vi "AI_StreamingAI_Save_Read.vi"() -> ()   [LabVIEW 2012]
panel:
  out "overrun count":i32
  in  "read buffer size":u64=131072
  in  "convert rate":dbl=1000000.0
  in  "channel count":i32=2
  in  "y min":dbl
  in  "y max":dbl=10.0
  in  "time out(s)":i32=10 caption="time out(10s)"
  out "Acquisition Szie":u64
  out "waveform chart":waveform(dbl)[](graph)
  in  "Disable Buffering? (T)":bool=TRUE caption="禁用缓冲？(T)"
  in  "number of samples per channel to read":u64=131072
  in  "File Path":path=path "c:/labview/data/data.tdms"
  in  "convert clock rate":dbl=1000000.0
  in  "start acq":bool
  in  "stop acq":bool
  in  "stop read":bool
  in  "read flag":bool
  in  "acq flag":bool
  in  "start read":bool
  in  "exist":bool
  # "Please modify physical channels and value range in Channel Parameters through DAQNavi Property Assistant VI  in block diagram.\nPlease modify the file path before save/read data.\nPlease modify the parameters in replay mode as actual value before Read&Display."
  # "Acquisition"
  # "Replay"
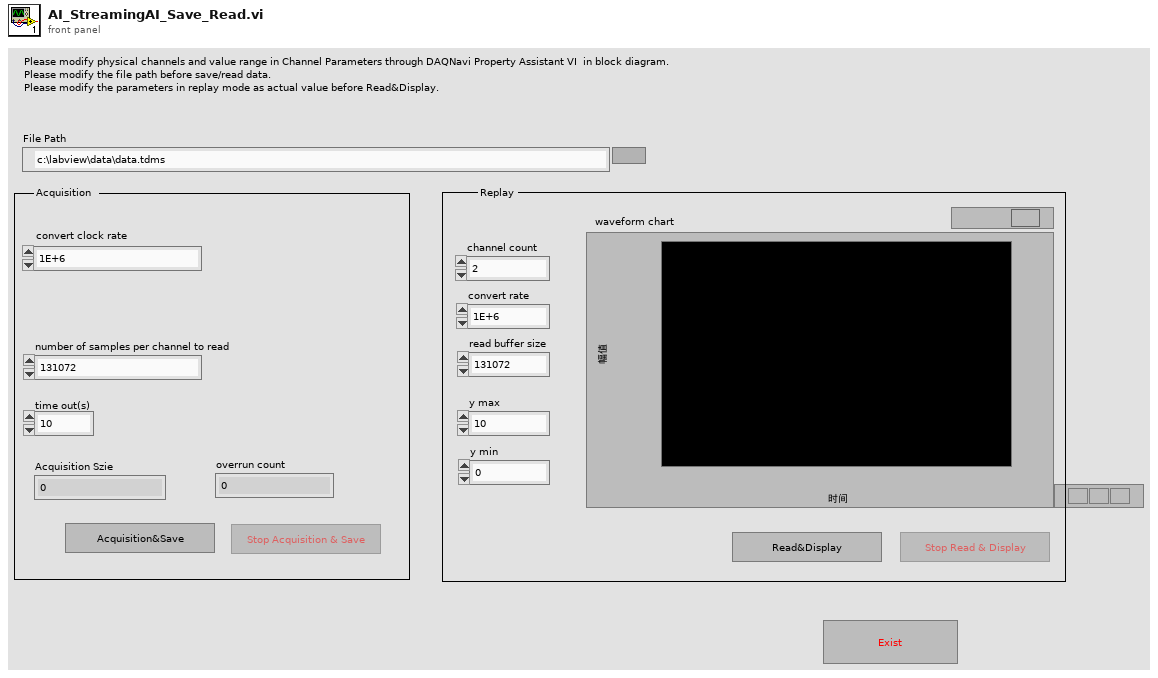
[diagram p1: front panel]
types:
  T1 = enum8{"Enabled", "Disabled", "Disabled and Grayed Out"}
  T2 = enum16{"open", "open or create", "create or replace", "create", "open (read-only)"}
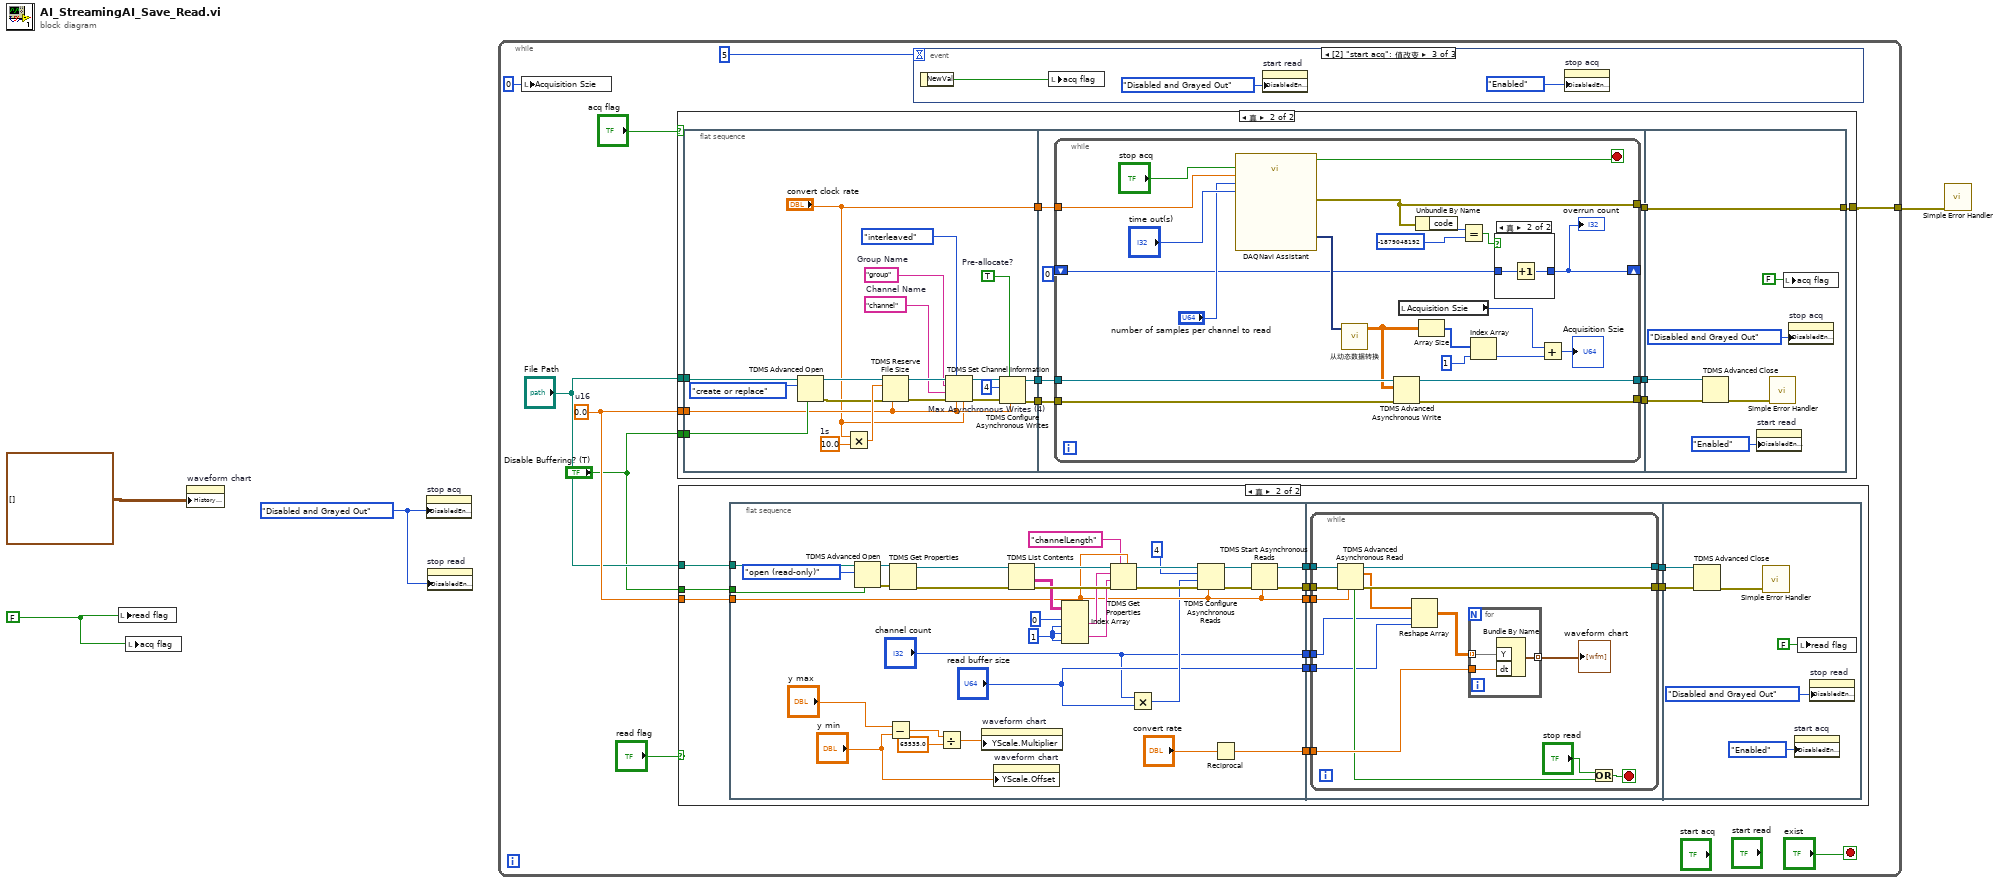
[diagram p0: block diagram]
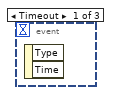
[diagram p5: hidden frame]
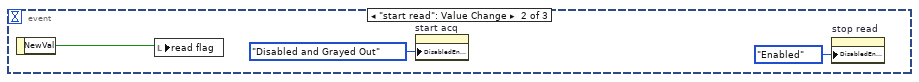
[diagram p6: hidden frame]
diagram:
  w3 = T1."Disabled and Grayed Out" ("禁用")
  w4 = FALSE ("read flag")
  n1 = local write "read flag"(w4) -> ()
  n2 = local write "acq flag"(w4) -> ()
  n3 = property on="waveform chart" class="WFChart (严格)"("History Data"=waveform(u16)[][] [] ("历史数据")) -> ()  [unwired: 2 in, 2 out]
  n4 = property on="stop acq" class="Bool"("DisabledEnum"=w3) -> ()  [unwired: 2 in, 2 out]
  n5 = property on="stop read" class="Bool"("DisabledEnum"=w3) -> ()  [unwired: 2 in, 2 out]
  n6 = while {
    tunnel: [w9] -> w1
    stop <- "exist" stop-if-true
    w8 = 0.0  # u16
    n7 = local write "Acquisition Szie"(0 ("Acquisition Szie")) -> ()
    n8 = case shown="真" "acq flag" {
      tunnel: "File Path" -> [_ w98]
      tunnel: [_ w92] -> w9
      tunnel: "Disable Buffering? (T)" -> [_ w91]
      tunnel: w8 -> [_ w90]
      frame False {
      }
      frame True {
        n9 = flat-sequence {
          tunnel: w98 -> [w107]
          tunnel: [w106] -> w97
          tunnel: [w105] -> w96
          tunnel: w91 -> [w104]
          tunnel: w90 -> [w103]
          tunnel: ["convert clock rate"] -> w89
          tunnel: w97 -> [w125]
          tunnel: w96 -> [w124]
          tunnel: [w123] -> w95
          tunnel: [w122] -> w94
          tunnel: [w121] -> w93
          tunnel: w89 -> [w120]
          tunnel: w95 -> [w156]
          tunnel: w94 -> [w155]
          tunnel: w93 -> [w154]
          tunnel: [w154] -> w92
          frame #0 {
            w102 = 10.0  # 1s
            w110 = "channel"  # Channel Name
            w111 = "group"  # Group Name
            w112 = u32 4  # Max Asynchronous Writes (4)
            w113 = TRUE  # Pre-allocate?
            n10 = TDMS Advanced Open(6:w104, 10:T2."create or replace" ("操作(0:open)"), 11:w107) -> (0:w100:errorcluster, 3:w101:refnum<k34>)  [unwired: 2 in, 1 out]
            n11 = Multiply(x="convert clock rate", y=w102) -> (x*y=w109:dbl)
            n12 = TDMS Reserve File Size(6:w103, 8:w100, 10:w109, 11:w101) -> (0:w117:errorcluster, 3:w116:refnum<k34>)  [unwired: 1 in]
            n13 = TDMS Set Channel Information(4:"convert clock rate", 6:w103, 7:enum16{"non-interleaved", "interleaved"}."interleaved" ("数据布局（0:非交叉）"), 8:w117, 9:w110, 10:w111, 11:w116) -> (0:w114:errorcluster, 3:w115:refnum<k34>)
            n14 = TDMS Configure Asynchronous Writes(6:w103, 7:w113, 8:w114, 10:w112, 11:w115) -> (0:w105:errorcluster, 3:w106:refnum<k34>)  [unwired: 2 in]
          }
          frame #1 {
            n15 = while {
              tunnel: w125 -> [w147]
              tunnel: w124 -> [w146]
              tunnel: [w145] -> w123
              tunnel: [w144] -> w122
              tunnel: [w133] -> w121
              tunnel: w120 -> [w140]
              shift-right: [w132] -> _
              shift-left: 0 -> [w131]
              stop <- w138 stop-if-true
              n16 = call "DAQNavi Assistant"("stop(true)"="stop acq", "conversion rate(Hz)"=w140, "samples"="number of samples per channel to read", "time out(10s)"="time out(s)") -> ("error out"=w133:errorcluster, "data out(DDT)"=w142:dynamicdata, "stopped"=w138:bool)  [unwired: 2 in, 19 out]
              n17 = call "从动态数据转换"("Dynamic Data Type"=w142) -> ("Array"=w126:dbl[][])  [unwired: 3 in]
              n18 = TDMS Advanced Asynchronous Write(8:w146, 10:w126, 11:w147) -> (0:w144:errorcluster, 3:w145:refnum<k34>)
              n19 = local read "Acquisition Szie"() -> (w143:u64)
              n20 = Unbundle By Name(w133) -> ("code"=w135:i32)
              n21 = Array Size(array=w126) -> (size(s)=w129:i32[])
              n22 = Equal?(x=w135, y=-1879048192) -> (x = y?=w130:bool)
              n23 = Index Array(array=w129, index=u64 1 ("y")) -> (element=w127:i32)
              n24 = case shown="真" w130 {
                tunnel: w131 -> [w148 w150]
                tunnel: [w148 w149] -> w132
                frame False {
                }
                frame True {
                  n25 = Increment(x=w150) -> (x+1=w149:i32)
                }
              }
              "overrun count" <- w132
              n26 = Add(x=w143, y=w127) -> (x+y=→"Acquisition Szie":u64)
            }
          }
          frame #2 {
            n27 = TDMS Advanced Close(8:w155, 11:w156) -> (0:w151:errorcluster)  [unwired: 2 in, 1 out]
            n28 = property on="start read" class="Bool"("DisabledEnum"=T1."Enabled" ("禁用")) -> ()  [unwired: 2 in, 2 out]
            n29 = call <vilib>:"Simple Error Handler.vi"("error in (no error)"=w151) -> ()  [unwired: 4 in, 5 out]
            n30 = local write "acq flag"(FALSE ("acq flag")) -> ()
            n31 = property on="stop acq" class="Bool"("DisabledEnum"=T1."Disabled and Grayed Out" ("禁用")) -> ()  [unwired: 2 in, 2 out]
          }
        }
      }
    }
    n32 = case shown="真" "read flag" {
      tunnel: "File Path" -> [_ w24]
      tunnel: "Disable Buffering? (T)" -> [_ w23]
      tunnel: w8 -> [_ w22]
      frame False {
      }
      frame True {
        n33 = flat-sequence {
          tunnel: w24 -> [w57]
          tunnel: w23 -> [w55]
          tunnel: w22 -> [w40]
          tunnel: [w44] -> w21
          tunnel: [w41] -> w20
          tunnel: [w40] -> w19
          tunnel: [w34] -> w18
          tunnel: ["channel count"] -> w15
          tunnel: ["read buffer size"] -> w14
          tunnel: w21 -> [w65]
          tunnel: w20 -> [w64]
          tunnel: w19 -> [w63]
          tunnel: w18 -> [w62]
          tunnel: [w61] -> w17
          tunnel: [w60] -> w16
          tunnel: w15 -> [w59]
          tunnel: w14 -> [w58]
          tunnel: w17 -> [w87]
          tunnel: w16 -> [w86]
          frame #0 {
            w48 = 1 ("禁用的索引 (列)")
            n34 = TDMS Advanced Open(6:w55, 10:T2."open (read-only)" ("操作(0:open)"), 11:w57) -> (0:w37:errorcluster, 3:w38:refnum<k34>)  [unwired: 2 in, 1 out]
            n35 = Subtract(x="y max", y="y min") -> (x-y=w30:dbl)
            n36 = TDMS Get Properties(8:w37, 11:w38) -> (0:w35:errorcluster, 3:w36:refnum<k34>)  [unwired: 4 in, 4 out]
            n37 = Divide(x=w30, y=65535.0) -> (x/y=w28:dbl)
            n38 = property on="waveform chart" class="WFChart (严格)"("YScale.Multiplier"=w28) -> ()  [unwired: 2 in, 2 out]
            n39 = property on="waveform chart" class="WFChart (严格)"("YScale.Offset"="y min") -> ()  [unwired: 2 in, 2 out]
            n40 = TDMS List Contents(4:w35, 7:w36) -> (0:w54:errorcluster, 1:w50:string[][], 3:w52:refnum<k34>)  [unwired: 1 in, 1 out]
            n41 = Index Array(array=w50, index (row) #1=0 ("索引 (行)"), index (col) #1=w48, index (row) #2=w48, index (col) #2=w48) -> (element #1=w47:string, element #2=w46:string)
            n42 = TDMS Get Properties(5:w40, 7:"channelLength" ("属性名称"), 8:w54, 9:w46, 10:w47, 11:w52) -> (0:w53:errorcluster, 3:w51:refnum<k34>)  [unwired: 4 out]
            n43 = Multiply(x="channel count", y="read buffer size") -> (x*y=w33:u64)
            n44 = TDMS Configure Asynchronous Reads(6:w40, 8:w53, 9:w33, 10:u32 4 ("缓冲区数量(4)"), 11:w51) -> (0:w42:errorcluster, 3:w43:refnum<k34>)  [unwired: 1 in]
            n45 = Reciprocal(x="convert rate") -> (1/x=w34:dbl)
            n46 = TDMS Start Asynchronous Reads(6:w40, 8:w42, 11:w43) -> (0:w41:errorcluster, 3:w44:refnum<k34>)  [unwired: 1 in]
          }
          frame #1 {
            n47 = while {
              tunnel: w65 -> [w79]
              tunnel: w64 -> [w78]
              tunnel: w63 -> [w77]
              tunnel: w62 -> [w75]
              tunnel: [w74] -> w61
              tunnel: [w73] -> w60
              tunnel: w59 -> [w67]
              tunnel: w58 -> [w68]
              stop <- w76 stop-if-true
              n48 = TDMS Advanced Asynchronous Read(6:w77, 8:w78, 11:w79) -> (0:w73:errorcluster, 2:w70:dbl[], 3:w74:refnum<k34>, 4:w72:bool)
              n49 = Reshape Array(w70, w67, w68) -> (w66:dbl[][])
              n50 = for {
                tunnel: [w82] -> w69 mode=indexing
                tunnel: w75 -> [w81]
                tunnel: w66 -> [w80] mode=indexing
                n51 = Bundle By Name("Y"=w80, "dt"=w81) -> (w82:waveform(dbl))  [unwired: 1 in]
              }
              "waveform chart" <- w69
              n52 = Or(x="stop read", y=w72) -> (x .or. y?=w76:bool)
            }
          }
          frame #2 {
            n53 = TDMS Advanced Close(8:w86, 11:w87) -> (0:w83:errorcluster)  [unwired: 2 in, 1 out]
            n54 = call <vilib>:"Simple Error Handler.vi"("error in (no error)"=w83) -> ()  [unwired: 4 in, 5 out]
            n55 = property on="start acq" class="Bool"("DisabledEnum"=T1."Enabled" ("禁用")) -> ()  [unwired: 2 in, 2 out]
            n56 = local write "read flag"(FALSE ("read flag")) -> ()
            n57 = property on="stop read" class="Bool"("DisabledEnum"=T1."Disabled and Grayed Out" ("禁用")) -> ()  [unwired: 2 in, 2 out]
          }
        }
      }
    }
    n58 = event shown="[2] \"start acq\": 值改变" {
      selector: _ -> [_ _ _]
      dyn-events: _ -> [_ _ _]
      timeout: 5 -> [_ _ _]
      event Timeout {
        n59 = event-data() -> ()  [unwired: 1 in, 2 out]
      }
      event "start read": Value Change {
        n60 = event-data() -> ("NewVal"=w160:bool)  [unwired: 1 in]
        n61 = local write "read flag"(w160) -> ()
        n62 = property on="start acq" class="Bool"("DisabledEnum"=T1."Disabled and Grayed Out" ("禁用")) -> ()  [unwired: 2 in, 2 out]
        n63 = property on="stop read" class="Bool"("DisabledEnum"=T1."Enabled" ("禁用")) -> ()  [unwired: 2 in, 2 out]
      }
      event "start acq": Value Change {
        n64 = event-data() -> ("NewVal"=w163:bool)  [unwired: 1 in]
        n65 = local write "acq flag"(w163) -> ()
        n66 = property on="start read" class="Bool"("DisabledEnum"=T1."Disabled and Grayed Out" ("禁用")) -> ()  [unwired: 2 in, 2 out]
        n67 = property on="stop acq" class="Bool"("DisabledEnum"=T1."Enabled" ("禁用")) -> ()  [unwired: 2 in, 2 out]
      }
    }
  }
  n68 = call <vilib>:"Simple Error Handler.vi"("error in (no error)"=w1) -> ()  [unwired: 4 in, 5 out]
